vi "Enqueue-execution.vi"(8 "error in (no error)":errorcluster, 9 "Timeout (ms)":i32=-1, 10 "Execution action":T1=enum."Execute sequence", 11 "State queue in":T2) -> (0 "error out":errorcluster, 1 "Timed out?":bool, 3 "State queue out":T2)   [LabVIEW 2013, in "PowderDeposition.lvlib" / "PD-Main.lvclass"]
doc: "Use this template to build a VI to use as a subVI."
uses:
  PD-Main.lvclass
  Object-reference.ctl
  Execution-actions.ctl
  PD-Main.lvclass/PD-Main.ctl
  Read Execution queue.vi
  Read Status.vi
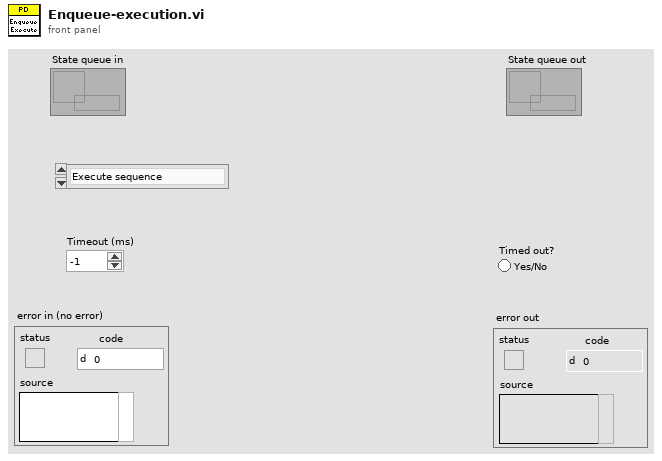
[diagram p1: front panel]
types:
  T1 = typedef "PowderDeposition.lvlib/PD-Main.lvclass/Execution-actions.ctl" = enum16{"Idle", "Execute action", "Execute sequence", "Execute seq with assert", "Exit"}
  T2 = typedef "PowderDeposition.lvlib/PD-Main.lvclass/Object-reference.ctl" = refnum<data-value>
  T3 = typedef "PowderDeposition.lvlib/PD-Data.lvclass/Statusses.ctl" = enum16{"Idle", "Initialized", "Configured", "Activated", "Started", "Paused", "Stopped", "Reset", "Error", "Exited"}
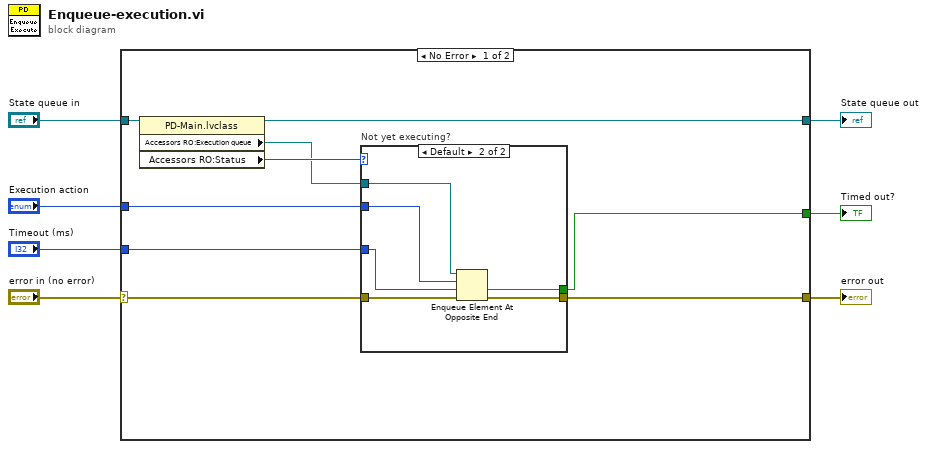
[diagram p0: block diagram]
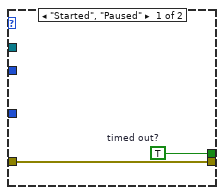
[diagram p2: hidden frame]
diagram:
  n1 = case shown="No Error" "error in (no error)" {
    selector: "error in (no error)" -> [w13 w26]
    tunnel: [w12 w26] -> w6
    tunnel: "Execution action" -> [w11 _]
    tunnel: "State queue in" -> [w16 w25]
    tunnel: [w15 w25] -> w4
    tunnel: "Timeout (ms)" -> [w10 _]
    tunnel: [w8 _] -> w2
    frame No Error {
      n2 = property class="PD-Main.lvclass"(reference=w16) -> (reference out=w15:T2, "Accessors RO:Execution queue"=w9:refnum<queue>, "Accessors RO:Status"=w14:T3)  [unwired: 1 in, 1 out]
      n3 = case "Not yet executing?" shown="Default" w14 {
        tunnel: w13 -> [w18 w24]
        tunnel: [w18 w23] -> w12
        tunnel: w11 -> [_ w20]
        tunnel: w10 -> [_ w19]
        tunnel: w9 -> [_ w21]
        tunnel: [w17 w22] -> w8
        frame "Started", "Paused" {
          w17 = TRUE  # timed out?
        }
        frame Default {
          n4 = Enqueue Element At Opposite End(queue=w21, element=w20, timeout in ms (-1)=w19, error in (no error)=w24) -> (timed out?=w22:bool, error out=w23:errorcluster)  [unwired: 1 out]
        }
      }
    }
    frame Error {
    }
  }
  "error out" <- w6
  "State queue out" <- w4
  "Timed out?" <- w2
